vi "4155C Transfer Config SMUs v3.0.vi"(0 "VISA resource name in":refnum<visa-resource-name>, 1 "Pulse period":dbl=0.005 min=0.005 max=1.0 step=0.0001 format="%.4f", 2 "Source/Common":u32(ring) items=["SMU1  ", "SMU2  ", "SMU3  ", "SMU4  ", "SMU5  ", "SMU6  ", "VSU1  ", "VSU2  "], 3 "Pulse width":dbl=0.0005 min=0.0005 max=0.1 step=0.0001 format="%.4f", 4 "Base voltage":dbl format="%^.4e", 5 "error in (no error)":errorcluster, 6 "sweep method":u16(ring) items=["Continuous", "Pulsed"], 7 "Probe 4":cluster{"on/off":bool, "Voltage":dbl} {"Voltage" min=-100.0 max=100.0 format="%.2f"}, 8 "Drain":u32(ring)=1 items=["SMU1  ", "SMU2  ", "SMU3  ", "SMU4  ", "SMU5  ", "SMU6  ", "VSU1  ", "VSU2  "], 9 "Gate":u32(ring)=2 items=["SMU1  ", "SMU2  ", "SMU3  ", "SMU4  ", "SMU5  ", "SMU6  ", "VSU1  ", "VSU2  "], 10 "Gate mode":u16(ring) items=["Auto", "Limited", "Fixed"], 11 "Source/drain mode":u16(ring) items=["Auto", "Limited", "Fixed"], 12 "Gate Range":u8(slide)=6 max=11 scale=0.0..11.0, 13 "Source/drain Range":u8(slide)=6 max=11 scale=0.0..11.0, 15 "Probe 4":u32(ring)=3 items=["SMU1  ", "SMU2  ", "SMU3  ", "SMU4  ", "SMU5  ", "SMU6  ", "VSU1  ", "VSU2  "], 17 "Drain Standby":bool, 18 "Gate Standby":bool) -> (14 "VISA Resource Name out":refnum<visa-resource-name>, 19 "error out":errorcluster)   [LabVIEW 2016]
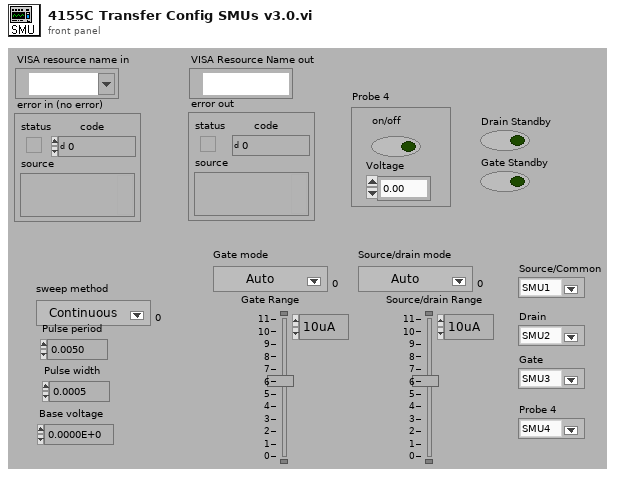
[diagram p1: front panel]
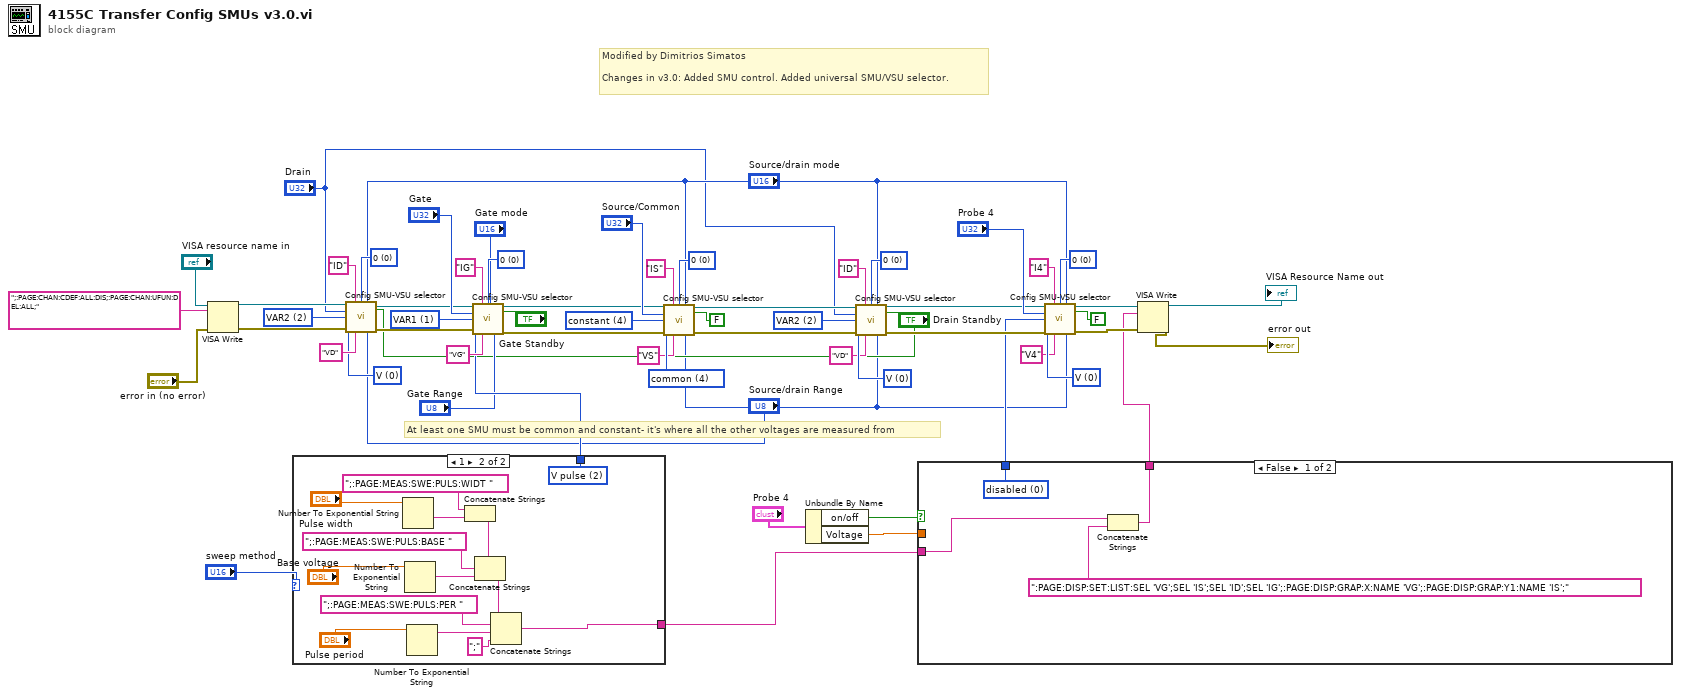
[diagram p0: block diagram]
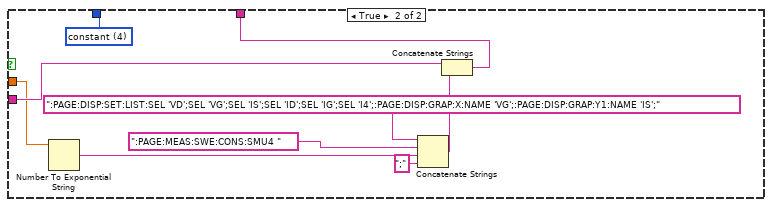
[diagram p2: hidden frame]
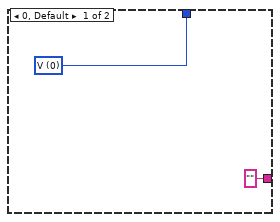
[diagram p3: hidden frame]
diagram:
  w19 = u32 2 items=["disabled  ", "VAR1  ", "VAR2  ", "VAR1'  ", "constant  "] ("function")
  w21 = u32 0 items=["0  ", "10K Ohms  ", "100K Ohms  ", "1M Ohms  "] ("series resistance *")
  w22 = u32 0 items=["V  ", "I  ", "V pulse  ", "I pulse  ", "  common  "] ("mode")
  w40 = u32 0 items=["V  ", "I  ", "V pulse  ", "I pulse  ", "  common  "] ("mode")
  w41 = u32 0 items=["0  ", "10K Ohms  ", "100K Ohms  ", "1M Ohms  "] ("series resistance *")
  w46 = u32 0 items=["0  ", "10K Ohms  ", "100K Ohms  ", "1M Ohms  "] ("series resistance *")
  w16 = u32 1 items=["disabled  ", "VAR1  ", "VAR2  ", "VAR1'  ", "constant  "] ("function")
  w50 = u32 0 items=["V  ", "I  ", "V pulse  ", "I pulse  ", "  common  "] ("mode")
  w51 = u32 0 items=["0  ", "10K Ohms  ", "100K Ohms  ", "1M Ohms  "] ("series resistance *")
  w53 = u32 2 items=["disabled  ", "VAR1  ", "VAR2  ", "VAR1'  ", "constant  "] ("function")
  w56 = u32 4 items=["V  ", "I  ", "V pulse  ", "I pulse  ", "  common  "] ("mode")
  w57 = u32 0 items=["0  ", "10K Ohms  ", "100K Ohms  ", "1M Ohms  "] ("series resistance *")
  w59 = u32 4 items=["disabled  ", "VAR1  ", "VAR2  ", "VAR1'  ", "constant  "] ("function")
  # "Modified by Dimitrios Simatos\n\nChanges in v3.0: Added SMU control. Added universal SMU/VSU selector."
  # "At least one SMU must be common and constant- it's where all the other voltages are measured from"
  n1 = VISA Write(VISA resource name="VISA resource name in", write buffer=";:PAGE:CHAN:CDEF:ALL:DIS;:PAGE:CHAN:UFUN:DEL:ALL;", error in (no error)="error in (no error)") -> (VISA resource name out=w4:refnum<visa-resource-name>, error out=w2:errorcluster)  [unwired: 1 out]
  n2 = case shown="1" "sweep method" {
    tunnel: [w62 w76] -> w30
    tunnel: ["" w64] -> w15
    frame 0, Default {
      w62 = u32 0 items=["V  ", "I  ", "V pulse  ", "I pulse  ", "  common  "] ("mode")
    }
    frame 1 {
      w76 = u32 2 items=["V  ", "I  ", "V pulse  ", "I pulse  ", "  common  "] ("mode")
      n3 = Number To Exponential String(number="Pulse width") -> (E-format string=w72:string)  [unwired: 3 in]
      n4 = Number To Exponential String(number="Base voltage") -> (E-format string=w68:string)  [unwired: 3 in]
      n5 = Number To Exponential String(number="Pulse period") -> (E-format string=w65:string)  [unwired: 3 in]
      n6 = Concatenate Strings(";:PAGE:MEAS:SWE:PULS:WIDT " ("Substring"), w72) -> (w70:string)
      n7 = Concatenate Strings(w70, ";:PAGE:MEAS:SWE:PULS:BASE " ("Substring"), w68) -> (w66:string)
      n8 = Concatenate Strings(w66, ";:PAGE:MEAS:SWE:PULS:PER " ("Substring"), w65, ";" ("Substring")) -> (w64:string)
    }
  }
  n9 = call "Config SMU-VSU selector.vi"("VISA session"=w4, "I name (max 6 chars)"="ID", "standby"="Drain Standby", "Range mode"="Source/drain mode", "unit to configure"="Drain", "function"=w19, "mode"=w22, "error in (no error)"=w2, "V name (max 6 chars)"="VD", "series resistance *"=w21, "Range"="Source/drain Range") -> ("dup VISA resource name"=w17:refnum<visa-resource-name>, "error out"=w18:errorcluster)  [unwired: 1 in, 2 out]
  n10 = call "Config SMU-VSU selector.vi"("VISA session"=w17, "I name (max 6 chars)"="IG", "standby"="Gate Standby", "Range mode"="Gate mode", "unit to configure"="Gate", "function"=w16, "mode"=w30, "error in (no error)"=w18, "V name (max 6 chars)"="VG", "series resistance *"=w46, "Range"="Gate Range") -> ("dup VISA resource name"=w27:refnum<visa-resource-name>, "error out"=w26:errorcluster)  [unwired: 1 in, 2 out]
  n11 = call "Config SMU-VSU selector.vi"("VISA session"=w27, "I name (max 6 chars)"="IS", "standby"=FALSE, "Range mode"="Source/drain mode", "unit to configure"="Source/Common", "function"=w59, "mode"=w56, "error in (no error)"=w26, "V name (max 6 chars)"="VS", "series resistance *"=w57, "Range"="Source/drain Range") -> ("dup VISA resource name"=w37:refnum<visa-resource-name>, "error out"=w36:errorcluster)  [unwired: 1 in, 2 out]
  n12 = Unbundle By Name("Probe 4") -> ("on/off"=w13:bool, "Voltage"=w14:dbl)
  n13 = call "Config SMU-VSU selector.vi"("VISA session"=w37, "I name (max 6 chars)"="ID", "standby"="Drain Standby", "Range mode"="Source/drain mode", "unit to configure"="Drain", "function"=w53, "mode"=w50, "error in (no error)"=w36, "V name (max 6 chars)"="VD", "series resistance *"=w51, "Range"="Source/drain Range") -> ("dup VISA resource name"=w24:refnum<visa-resource-name>, "error out"=w25:errorcluster)  [unwired: 1 in, 2 out]
  n14 = case shown="False" w13 {
    tunnel: w15 -> [w79 w89]
    tunnel: [w78 w88] -> w11
    tunnel: w14 -> [_ w86]
    tunnel: [w77 w87] -> w10
    frame False {
      w77 = u32 0 items=["disabled  ", "VAR1  ", "VAR2  ", "VAR1'  ", "constant  "] ("function")
      n15 = Concatenate Strings(w79, ":PAGE:DISP:SET:LIST:SEL 'VG';SEL 'IS';SEL 'ID';SEL 'IG';:PAGE:DISP:GRAP:X:NAME 'VG';:PAGE:DISP:GRAP:Y1:NAME 'IS';" ("write buffer (\"\")")) -> (w78:string)
    }
    frame True {
      w87 = u32 4 items=["disabled  ", "VAR1  ", "VAR2  ", "VAR1'  ", "constant  "] ("function")
      n16 = Number To Exponential String(number=w86) -> (E-format string=w84:string)  [unwired: 3 in]
      n17 = Concatenate Strings(":PAGE:DISP:SET:LIST:SEL 'VD';SEL 'VG';SEL 'IS';SEL 'ID';SEL 'IG';SEL 'I4';:PAGE:DISP:GRAP:X:NAME 'VG';:PAGE:DISP:GRAP:Y1:NAME 'IS';" ("write buffer (\"\")"), ":PAGE:MEAS:SWE:CONS:SMU4 " ("write buffer (\"\")"), w84, ";" ("Substring")) -> (w82:string)
      n18 = Concatenate Strings(w89, w82) -> (w88:string)
    }
  }
  n19 = call "Config SMU-VSU selector.vi"("VISA session"=w24, "I name (max 6 chars)"="I4", "standby"=FALSE, "Range mode"="Source/drain mode", "unit to configure"="Probe 4", "function"=w10, "mode"=w40, "error in (no error)"=w25, "V name (max 6 chars)"="V4", "series resistance *"=w41, "Range"="Source/drain Range") -> ("dup VISA resource name"=w35:refnum<visa-resource-name>, "error out"=w34:errorcluster)  [unwired: 1 in, 2 out]
  n20 = VISA Write(VISA resource name=w35, write buffer=w11, error in (no error)=w34) -> (VISA resource name out=→"VISA Resource Name out":refnum<visa-resource-name>, error out=→"error out":errorcluster)  [unwired: 1 out]
